vi "SPE XML Parse v1.0.vi"(7 "Error In":errorcluster, 10 "XML String":string) -> (0 "Error Out":errorcluster, 1 "Parse Errors":string, 3 "DataBlock Info":T1)   [LabVIEW 2015]
uses:
  <vilib>/xml/Close Reference(Node).vi
  <vilib>/xml/Close Reference(NNMap).vi
  <vilib>/xml/NI_XML.lvlib
  <resource>/objmgr/DOMUserDefRef.rc
panel:
  out "ROI error out":errorcluster
  out "N ROI":i64
  out "ROI widths":i64[](array[numeric])
  out "ROI heights":i64[](array[numeric])
  out "ROI strides":i64[](array[numeric])
  out "ROI sizes":i64[](array[numeric])
  out "frame stride":i64
  out "frame size":i64
  out "frame count":i64
  out "XML":string
  # "ROI Error note:\nDue to the way that NI coded the Next Non-Text Sibling.vi it will often throw error -2630. This is only a problem when there is more than 1 ROI per frame"
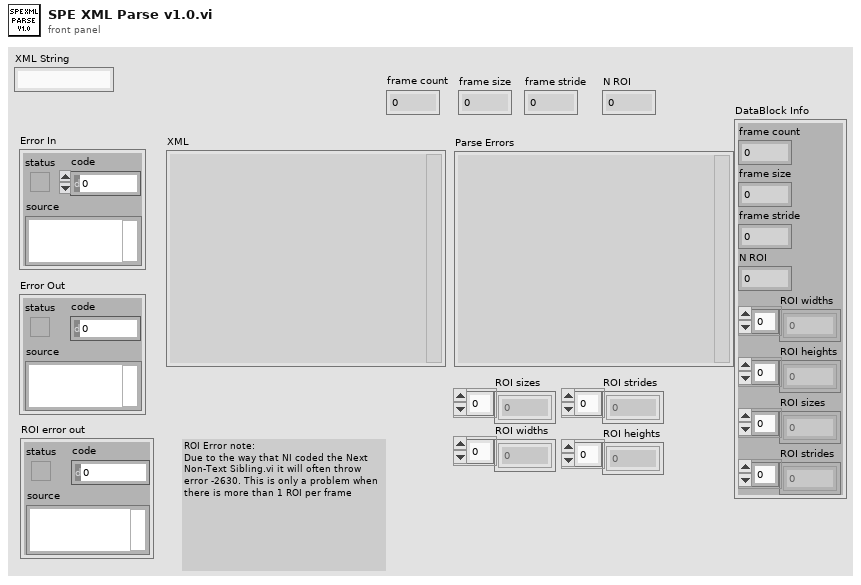
[diagram p1: front panel]
types:
  T1 = cluster{"frame count":i64, "frame size":i64, "frame stride":i64, "N ROI":i64, "ROI widths":i64[], "ROI heights":i64[], "ROI sizes":i64[], "ROI strides":i64[]}
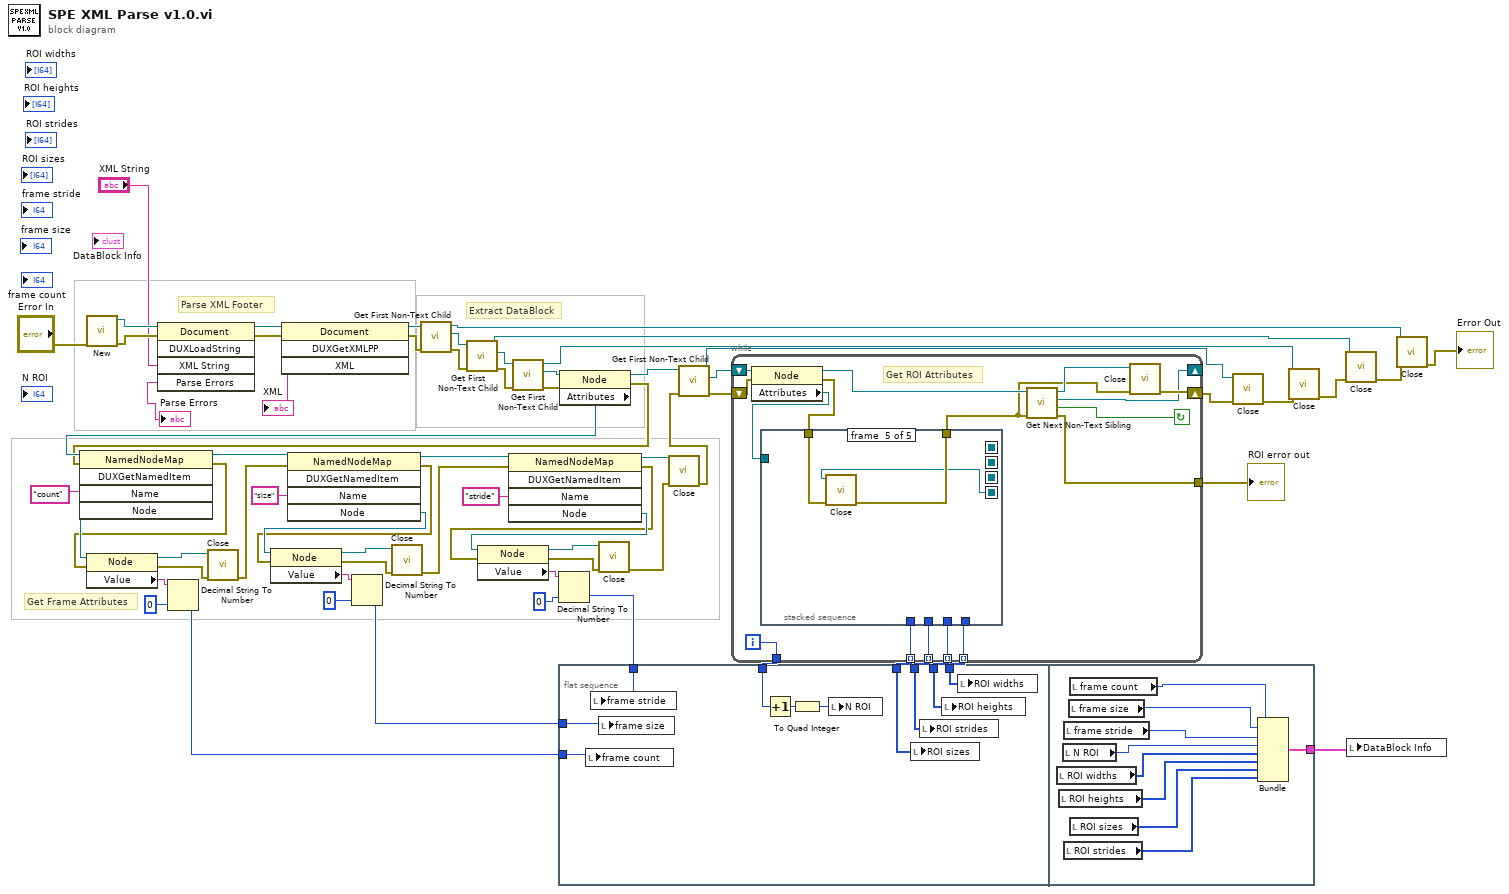
[diagram p0: block diagram]
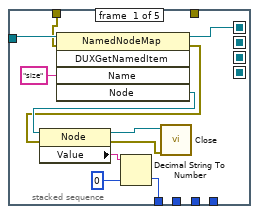
[diagram p2: hidden frame]
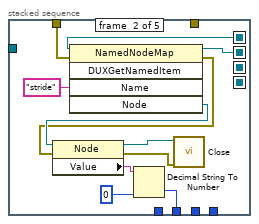
[diagram p3: hidden frame]
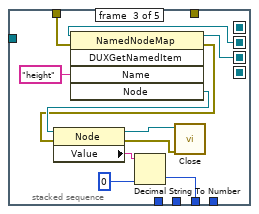
[diagram p4: hidden frame]
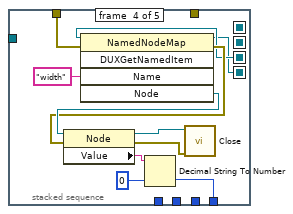
[diagram p5: hidden frame]
diagram:
  # "Get Frame Attributes"
  # "Extract DataBlock"
  # "Parse XML Footer"
  n1 = call <vilib>:"New.vi"("error in (no error)"="Error In") -> ("error out"=w64:errorcluster, "DOM document out"=w63:refnum<k20>)  [unwired: 7 in]
  n2 = invoke class="Document" method="DUXLoadString"(reference=w63, error in=w64, "XML String"="XML String") -> (reference out=w62:refnum<k20>, error out=w61:errorcluster, "Parse Errors"=→"Parse Errors":string)  [unwired: 2 in, 2 out]
  n3 = invoke class="Document" method="DUXGetXMLPP"(reference=w62, error in=w61) -> (reference out=w66:refnum<k20>, error out=w65:errorcluster, "XML"=→"XML":string)  [unwired: 2 in, 1 out]
  n4 = call <vilib>:"Get First Non-Text Child.vi"("error in (no error)"=w65, "node in"=w66) -> ("error out"=w57:errorcluster, "child node"=w58:refnum<k20>, "node out"=w59:refnum<k20>)  [unwired: 6 in, 1 out]
  n5 = call <vilib>:"Get First Non-Text Child.vi"("error in (no error)"=w57, "node in"=w58) -> ("error out"=w53:errorcluster, "child node"=w54:refnum<k20>, "node out"=w56:refnum<k20>)  [unwired: 6 in, 1 out]
  n6 = call <vilib>:"Get First Non-Text Child.vi"("error in (no error)"=w53, "node in"=w54) -> ("error out"=w45:errorcluster, "child node"=w46:refnum<k20>, "node out"=w52:refnum<k20>)  [unwired: 6 in, 1 out]
  n7 = flat-sequence {
    tunnel: w17 -> [w78]
    tunnel: w16 -> [w77]
    tunnel: w15 -> [w76]
    tunnel: w14 -> [w75]
    tunnel: w13 -> [w74]
    tunnel: w12 -> [w73]
    tunnel: w11 -> [w72]
    tunnel: w10 -> [w71]
    tunnel: [w79] -> w2
    frame #0 {
      n8 = local write "frame count"(w74) -> ()
      n9 = local write "frame stride"(w72) -> ()
      n10 = local write "frame size"(w73) -> ()
      n11 = Increment(x=w71) -> (x+1=w70:i32)
      n12 = To Quad Integer(1:w70) -> (0:w69:i64)
      n13 = local write "N ROI"(w69) -> ()
      n14 = local write "ROI sizes"(w78) -> ()
      n15 = local write "ROI strides"(w77) -> ()
      n16 = local write "ROI heights"(w76) -> ()
      n17 = local write "ROI widths"(w75) -> ()
    }
    frame #1 {
      n18 = local read "ROI widths"() -> (w83:i64[])
      n19 = local read "ROI heights"() -> (w82:i64[])
      n20 = local read "N ROI"() -> (w84:i64)
      n21 = local read "frame stride"() -> (w85:i64)
      n22 = local read "ROI strides"() -> (w80:i64[])
      n23 = local read "frame size"() -> (w86:i64)
      n24 = local read "frame count"() -> (w87:i64)
      n25 = local read "ROI sizes"() -> (w81:i64[])
      n26 = Bundle("frame count"=w87, "frame size"=w86, "frame stride"=w85, "N ROI"=w84, "ROI widths"=w83, "ROI heights"=w82, "ROI sizes"=w81, "ROI strides"=w80) -> (w79:T1)  [unwired: 1 in]
    }
  }
  n27 = property class="Node"(reference=w46, error in=w45) -> (reference out=w22:refnum<k20>, error out=w44:errorcluster, "Attributes"=w49:refnum<k20>)
  n28 = invoke class="NamedNodeMap" method="DUXGetNamedItem"(reference=w49, error in=w44, "Name"="count") -> (reference out=w41:refnum<k20>, error out=w40:errorcluster, "Node"=w48:refnum<k20>)  [unwired: 2 in, 2 out]
  n29 = property class="Node"(reference=w48, error in=w40) -> (reference out=w47:refnum<k20>, error out=w42:errorcluster, "Value"=w43:string)
  n30 = Decimal String To Number(string=w43, default (0L)=i64 0) -> (number=w13:i64)  [unwired: 1 in, 1 out]
  n31 = call-poly <vilib>:"Close.vi"("error in (no error)"=w42, "node"=w47) -> ("error out"=w39:errorcluster)  [unwired: 7 in]
  n32 = invoke class="NamedNodeMap" method="DUXGetNamedItem"(reference=w41, error in=w39, "Name"="size") -> (reference out=w37:refnum<k20>, error out=w32:errorcluster, "Node"=w33:refnum<k20>)  [unwired: 2 in, 2 out]
  n33 = property class="Node"(reference=w33, error in=w32) -> (reference out=w36:refnum<k20>, error out=w34:errorcluster, "Value"=w35:string)
  n34 = Decimal String To Number(string=w35, default (0L)=i64 0 ("default (0 I32)")) -> (number=w12:i64)  [unwired: 1 in, 1 out]
  n35 = call-poly <vilib>:"Close.vi"("error in (no error)"=w34, "node"=w36) -> ("error out"=w31:errorcluster)  [unwired: 7 in]
  n36 = invoke class="NamedNodeMap" method="DUXGetNamedItem"(reference=w37, error in=w31, "Name"="stride") -> (reference out=w24:refnum<k20>, error out=w25:errorcluster, "Node"=w26:refnum<k20>)  [unwired: 2 in, 2 out]
  n37 = property class="Node"(reference=w26, error in=w25) -> (reference out=w29:refnum<k20>, error out=w27:errorcluster, "Value"=w28:string)
  n38 = Decimal String To Number(string=w28, default (0L)=i64 0) -> (number=w11:i64)  [unwired: 1 in, 1 out]
  n39 = call-poly <vilib>:"Close.vi"("error in (no error)"=w27, "node"=w29) -> ("error out"=w23:errorcluster)  [unwired: 7 in]
  n40 = call-poly <vilib>:"Close.vi"("error in (no error)"=w23, "named node map"=w24) -> ("error out"=w21:errorcluster)  [unwired: 7 in]
  n41 = call <vilib>:"Get First Non-Text Child.vi"("error in (no error)"=w21, "node in"=w22) -> ("error out"=w19:errorcluster, "child node"=w18:refnum<k20>, "node out"=w9:refnum<k20>)  [unwired: 6 in, 1 out]
  n42 = while {
    shift-right: [w90] -> _
    shift-left: w18 -> [w103]
    shift-right: [w94] -> w8
    shift-left: w19 -> [w102]
    tunnel: [w100] -> w17 mode=indexing
    tunnel: [w99] -> w16 mode=indexing
    tunnel: [w98] -> w15 mode=indexing
    tunnel: [w97] -> w14 mode=indexing
    tunnel: [w96] -> w10
    tunnel: [w88] -> w1
    i -> [w96]
    stop <- w91 continue-if-true
    # "Get ROI Attributes"
    n43 = property class="Node"(reference=w103, error in=w102) -> (reference out=w92:refnum<k20>, error out=w101:errorcluster, "Attributes"=w95:refnum<k20>)
    n44 = stacked-sequence {
      seq-local: [w104 _ _ _ _] -> [_ w116 _ _ _]
      seq-local: [_ w115 _ _ _] -> [_ _ w127 _ _]
      seq-local: [_ _ w126 _ _] -> [_ _ _ w138 _]
      seq-local: [_ _ _ w137 _] -> [_ _ _ _ w148]
      tunnel: [w108 _ _ _ _] -> w100
      tunnel: w95 -> [w107 _ _ _ _]
      tunnel: w101 -> [w106 w119 w130 w141 w150]
      tunnel: [_ w118 _ _ _] -> w99
      tunnel: [_ _ w129 _ _] -> w98
      tunnel: [_ _ _ w140 _] -> w97
      tunnel: [_ _ _ _ w149] -> w89
      frame #0 {
        n45 = invoke class="NamedNodeMap" method="DUXGetNamedItem"(reference=w107, error in=w106, "Name"="size") -> (reference out=w104:refnum<k20>, error out=w109:errorcluster, "Node"=w110:refnum<k20>)  [unwired: 2 in, 2 out]
        n46 = property class="Node"(reference=w110, error in=w109) -> (reference out=w113:refnum<k20>, error out=w111:errorcluster, "Value"=w112:string)
        n47 = Decimal String To Number(string=w112, default (0L)=i64 0) -> (number=w108:i64)  [unwired: 1 in, 1 out]
        n48 = call-poly <vilib>:"Close.vi"("error in (no error)"=w111, "node"=w113) -> ()  [unwired: 7 in, 1 out]
      }
      frame #1 {
        n49 = invoke class="NamedNodeMap" method="DUXGetNamedItem"(reference=w116, error in=w119, "Name"="stride") -> (reference out=w115:refnum<k20>, error out=w120:errorcluster, "Node"=w121:refnum<k20>)  [unwired: 2 in, 2 out]
        n50 = property class="Node"(reference=w121, error in=w120) -> (reference out=w124:refnum<k20>, error out=w122:errorcluster, "Value"=w123:string)
        n51 = Decimal String To Number(string=w123, default (0L)=i64 0) -> (number=w118:i64)  [unwired: 1 in, 1 out]
        n52 = call-poly <vilib>:"Close.vi"("error in (no error)"=w122, "node"=w124) -> ()  [unwired: 7 in, 1 out]
      }
      frame #2 {
        n53 = invoke class="NamedNodeMap" method="DUXGetNamedItem"(reference=w127, error in=w130, "Name"="height") -> (reference out=w126:refnum<k20>, error out=w131:errorcluster, "Node"=w132:refnum<k20>)  [unwired: 2 in, 2 out]
        n54 = property class="Node"(reference=w132, error in=w131) -> (reference out=w135:refnum<k20>, error out=w133:errorcluster, "Value"=w134:string)
        n55 = Decimal String To Number(string=w134, default (0L)=i64 0) -> (number=w129:i64)  [unwired: 1 in, 1 out]
        n56 = call-poly <vilib>:"Close.vi"("error in (no error)"=w133, "node"=w135) -> ()  [unwired: 7 in, 1 out]
      }
      frame #3 {
        n57 = invoke class="NamedNodeMap" method="DUXGetNamedItem"(reference=w138, error in=w141, "Name"="width") -> (reference out=w137:refnum<k20>, error out=w142:errorcluster, "Node"=w143:refnum<k20>)  [unwired: 2 in, 2 out]
        n58 = property class="Node"(reference=w143, error in=w142) -> (reference out=w146:refnum<k20>, error out=w144:errorcluster, "Value"=w145:string)
        n59 = Decimal String To Number(string=w145, default (0L)=i64 0) -> (number=w140:i64)  [unwired: 1 in, 1 out]
        n60 = call-poly <vilib>:"Close.vi"("error in (no error)"=w144, "node"=w146) -> ()  [unwired: 7 in, 1 out]
      }
      frame #4 {
        n61 = call-poly <vilib>:"Close.vi"("error in (no error)"=w150, "named node map"=w148) -> ("error out"=w149:errorcluster)  [unwired: 7 in]
      }
    }
    n62 = call <vilib>:"Get Next Non-Text Sibling.vi"("error in (no error)"=w89, "node in"=w92) -> ("error out"=w88:errorcluster, "found sibling node?"=w91:bool, "sibling node"=w90:refnum<k20>, "node out"=w93:refnum<k20>)  [unwired: 6 in]
    n63 = call-poly <vilib>:"Close.vi"("error in (no error)"=w89, "node"=w93) -> ("error out"=w94:errorcluster)  [unwired: 7 in]
  }
  "ROI error out" <- w1
  n64 = call-poly <vilib>:"Close.vi"("error in (no error)"=w8, "node"=w9) -> ("error out"=w51:errorcluster)  [unwired: 7 in]
  n65 = call-poly <vilib>:"Close.vi"("error in (no error)"=w51, "node"=w52) -> ("error out"=w55:errorcluster)  [unwired: 7 in]
  n66 = call-poly <vilib>:"Close.vi"("error in (no error)"=w55, "node"=w56) -> ("error out"=w20:errorcluster)  [unwired: 7 in]
  n67 = local write "DataBlock Info"(w2) -> ()
  n68 = call-poly <vilib>:"Close.vi"("error in (no error)"=w20, "node"=w59) -> ("error out"=→"Error Out":errorcluster)  [unwired: 7 in]
